vi "PV ActiveLine relay switch point.vi"(8 "error in (no error)":errorcluster, 9 "PV ActiveLine relay switch point - Cluster":T1={"Parameter"=enum." Pressure Set Point 1 [hPa ; mbar] (730)", "Parameter\nread only<->describe"=FALSE, "Pressure switch point (hPa)"=1.0000000005} {"Pressure switch point (hPa)" min=5e-10 max=2000.0 step=1.0 format="%_3e"}, 10 "Adress of unit":u16=10 max=999 step=1, 11 "VISA session":refnum<visa-resource-name>) -> (0 "error out":errorcluster, 2 "response (data)":string, 3 "dup VISA session":refnum<visa-resource-name>)   [LabVIEW 2021, in "Pfeiffer Vacuum.lvlib"]
doc: "There are two parameters available, only one of which can be enabled at a time. \n\n0 - Pressure switch point 1 [mbar] (default) (730)\n1 - Pressure switch point 2 [mbar] (732)\n\nNote: The one control right of this one will set the appropriate values for the selected parameter. Any settings for an parameter that is not selected will be ignored. If a value is out of range, it will be changed to either the upper or the lower limit of the range."
uses:
  <instrlib>/Pfeiffer Vacuum/Pfeiffer Vacuum.lvlib
  <instrlib>/Pfeiffer Vacuum/Public/ActiveLine/PV ActiveLine relay switch point - Cluster.ctl
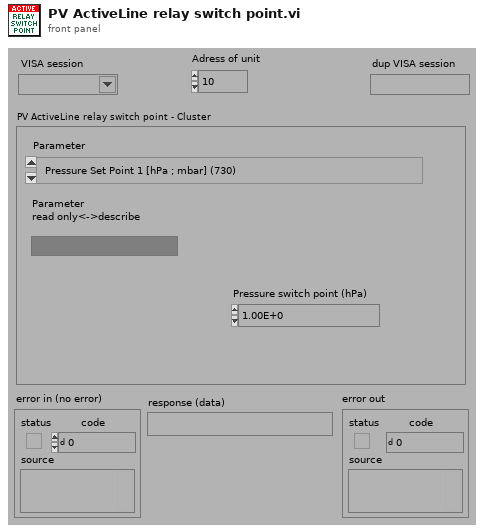
[diagram p1: front panel]
types:
  T1 = typedef "Pfeiffer Vacuum.lvlib/PV ActiveLine relay switch point - Cluster.ctl" = cluster{"Parameter":enum16{" Pressure Set Point 1 [hPa ; mbar] (730)", " Pressure Set Point 2 [hPa ; mbar] (732)"}, "Parameter\nread only<->describe":bool, "Pressure switch point (hPa)":dbl}
  T2 = enum16{" Pressure Set Point 1 [hPa ; mbar] (730)", " Pressure Set Point 2 [hPa ; mbar] (732)"}
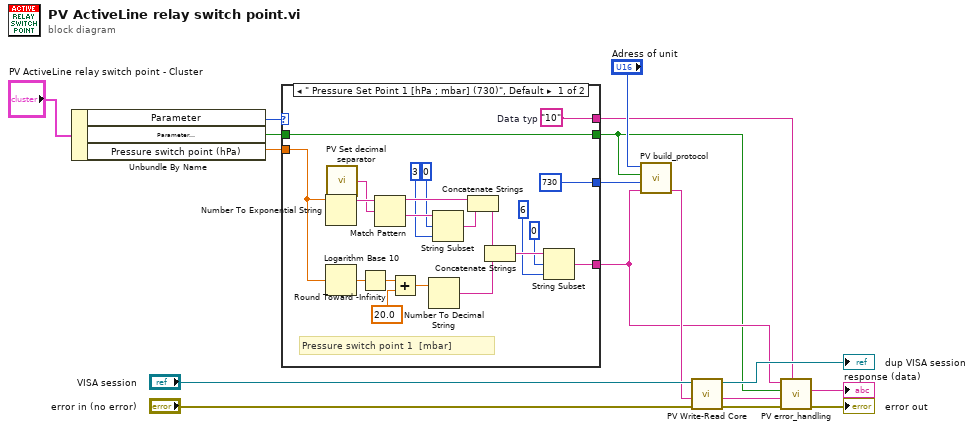
[diagram p0: block diagram]
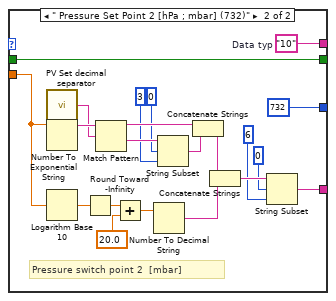
[diagram p2: hidden frame]
diagram:
  n1 = Unbundle By Name("PV ActiveLine relay switch point - Cluster") -> ("Parameter"=w15:T2, "Parameter\nread only<->describe"=w14:bool, "Pressure switch point (hPa)"=w2:dbl)
  n2 = case shown="\" Pressure Set Point 1 [hPa ; mbar] (730)\", Default" w15 {
    tunnel: [u16 730 ("Parameter-number") u16 732 ("Parameter-number")] -> w16
    tunnel: [w19 w40] -> w5
    tunnel: [w37 w58] -> w4
    tunnel: w14 -> [w37 w58]
    tunnel: w2 -> [w20 w41]
    tunnel: [w36 w57] -> w6
    frame " Pressure Set Point 1 [hPa ; mbar] (730)", Default {
      w36 = "10"  # Data typ
      # "Pressure switch point 1  [mbar]"
      n3 = Number To Exponential String(number=w20) -> (E-format string=w32:string)  [unwired: 3 in]
      n4 = Logarithm Base 10(1:w20) -> (0:w35:dbl)
      n5 = call <instrlib>:"PV Set decimal separator.vi"() -> ("decimal separator"=w18:string)
      n6 = Round Toward -Infinity(1:w35) -> (0:w34:dbl)
      n7 = Match Pattern(string=w32, regular expression=w18) -> (before substring=w33:string, after substring=w31:string)  [unwired: 1 in, 2 out]
      n8 = Add(x=w34, y=20.0) -> (x+y=w27:dbl)
      n9 = Number To Decimal String(number=w27) -> (decimal integer string=w24:string)  [unwired: 1 in]
      n10 = String Subset(string=w31, offset (0)=0 ("Offset (0)"), length (rest)=3 ("Länge")) -> (substring=w28:string)
      n11 = Concatenate Strings(w33, w28) -> (w25:string)
      n12 = Concatenate Strings(w25, w24) -> (w23:string)
      n13 = String Subset(string=w23, offset (0)=0 ("Offset (0)"), length (rest)=6 ("Länge")) -> (substring=w19:string)
    }
    frame " Pressure Set Point 2 [hPa ; mbar] (732)" {
      w57 = "10"  # Data typ
      # "Pressure switch point 2  [mbar]"
      n14 = call <instrlib>:"PV Set decimal separator.vi"() -> ("decimal separator"=w39:string)
      n15 = Number To Exponential String(number=w41) -> (E-format string=w53:string)  [unwired: 3 in]
      n16 = Logarithm Base 10(1:w41) -> (0:w56:dbl)
      n17 = Round Toward -Infinity(1:w56) -> (0:w55:dbl)
      n18 = Match Pattern(string=w53, regular expression=w39) -> (before substring=w54:string, after substring=w52:string)  [unwired: 1 in, 2 out]
      n19 = Add(x=w55, y=20.0) -> (x+y=w48:dbl)
      n20 = Number To Decimal String(number=w48) -> (decimal integer string=w45:string)  [unwired: 1 in]
      n21 = String Subset(string=w52, offset (0)=0 ("Offset (0)"), length (rest)=3 ("Länge")) -> (substring=w49:string)
      n22 = Concatenate Strings(w54, w49) -> (w46:string)
      n23 = Concatenate Strings(w46, w45) -> (w44:string)
      n24 = String Subset(string=w44, offset (0)=0 ("Offset (0)"), length (rest)=6 ("Länge")) -> (substring=w40:string)
    }
  }
  n25 = call <instrlib>:"PV build_protocol.vi"("Data"=w5, "Parameter-number"=w16, "parameter\nread<->describe"=w4, "Adress"="Adress of unit") -> ("output"=w10:string)  [unwired: 3 in]
  n26 = call <instrlib>:"PV Write-Read Core.vi"("error in"="error in (no error)", "Write data in"=w10, "VISA session"="VISA session") -> ("error out"=w7:errorcluster, "response (data) out"=w8:string, "dup VISA session"=→"dup VISA session":refnum<visa-resource-name>)  [unwired: 2 in]
  n27 = call <instrlib>:"PV error_handling.vi"("Data Typ in"=w6, "error in"=w7, "response (data) in"=w8, "Parameter\nread only<->describe"=w4, "data in"=w5) -> ("error out"=→"error out":errorcluster, "Data out"=→"response (data)":string)  [unwired: 4 in, 1 out]
